vi "showStatusText.vi"(8 "Error In":errorcluster, 10 "widget":refnum<class "QWidget.lvclass">, 11 "QAction In":refnum<class "QAction.lvclass">) -> (0 "Error Out":errorcluster, 2 "Value":bool, 3 "QAction Out":refnum<class "QAction.lvclass">)   [LabVIEW 2014, in "QAction.lvclass"]
doc: "LabVIEW-specific documentation is not yet available. See <b>http://doc.qt.io/qt-5/QAction.html#showStatusText</b>"
uses:
  QAction.lvclass
  QWidget/QWidget.lvclass
  LQ Core/LQIdentity/LQIdentity.lvclass/LQIdentity.ctl
  LQ Core/LQ Core.lvlib
  LQ Core/LQIdentity/LQIdentity.lvclass
panel:
  # "Copyright (c) 2016 Sze Howe Koh\n\nThis Source Code Form is subject to the terms of the Mozilla Public\nLicense, v. 2.0. If a copy of the MPL was not distributed with this\nfile, You can obtain one at http://mozilla.org/MPL/2.0/."
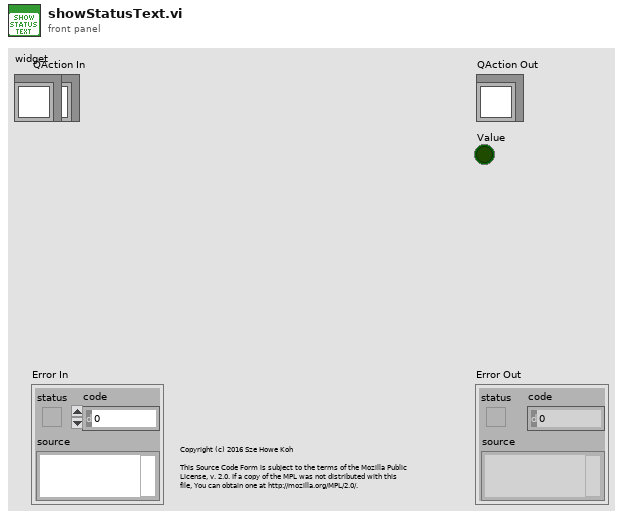
[diagram p1: front panel]
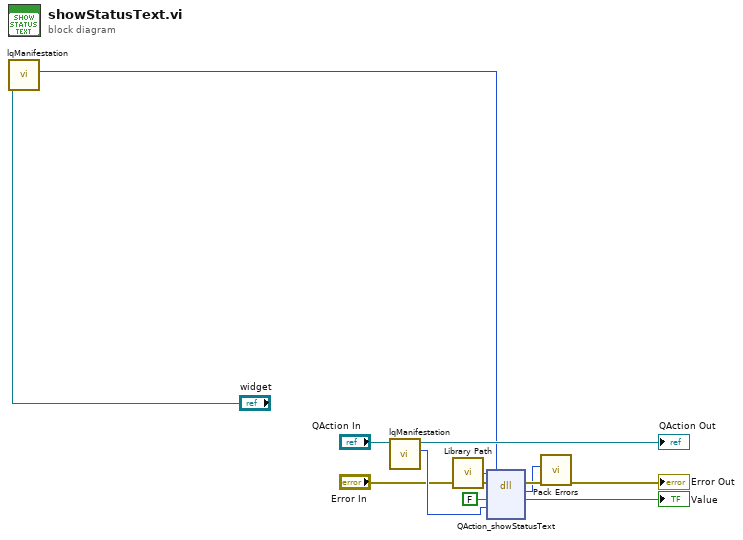
[diagram p0: block diagram]
diagram:
  n1 = call "lqManifestation.vi"("LQIdentity in"="widget") -> ("Manifestation"=w1:u64)  [unwired: 9 in, 1 out]
  n2 = call "lqManifestation.vi"("LQIdentity in"="QAction In") -> ("Manifestation"=w7:u64, "LQIdentity out"=→"QAction Out":refnum<class "QAction.lvclass">)  [unwired: 9 in]
  n3 = call "Library Path.vi"() -> ("Library Path"=w8:path)
  n4 = dll-call lib="?" fn="QAction_showStatusText"(path in=w8, error in="Error In", "_retVal"=FALSE, "_instance"=w7, "widget"=w1) -> (error out=w5:errorcluster, w3:i32, "_retVal"=→"Value":bool)  [unwired: 3 in, 1 out]
  n5 = call "Pack Errors.vi"("Error In"=w5, "Error Code"=w3) -> ("Error Out"=→"Error Out":errorcluster)  [unwired: 9 in]
